vi "Atividade 5.vi"() -> ()   [LabVIEW 2015]
panel:
  out "Numeric":dbl
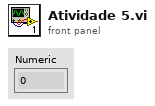
[diagram p1: front panel]
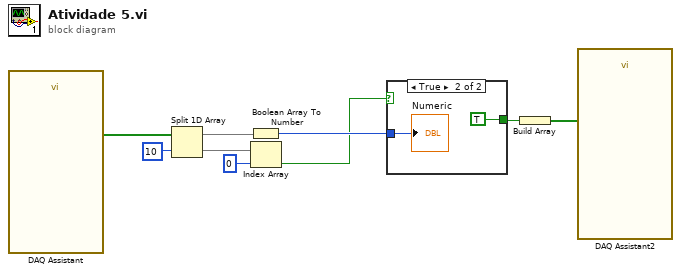
[diagram p0: block diagram]
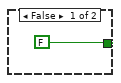
[diagram p2: hidden frame]
diagram:
  n1 = call "DAQ Assistant"() -> ("data"=w5:bool[])  [unwired: 17 in, 2 out]
  n2 = Split 1D Array(array=w5, index=10) -> (first subarray=w6:bool[], second subarray=w7:bool[])
  n3 = Boolean Array To Number(Boolean array=w6) -> (number=w9:u32)
  n4 = Index Array(array=w7, index=0) -> (element=w3:bool)
  n5 = case shown="True" w3 {
    tunnel: w9 -> [_ w12]
    tunnel: [FALSE TRUE] -> w2
    frame False {
    }
    frame True {
      "Numeric" <- w12
    }
  }
  n6 = Build Array(w2) -> (w1:bool[])
  n7 = call "DAQ Assistant2"("data"=w1) -> ()  [unwired: 17 in, 2 out]
